vi "PIM Convert 1.0 to 1.1.vi"(0 "PIM 1.0 Test Parameters":T2={"Step Tag"="", "Quickmode?"=FALSE, "PIM Test Stimulus"={"C1 Pwr dBm"=0.0, "C2 Pwr dBm"=0.0, "Power Units"=enum."dBm", "Meas Type"=enum."Band Edges", "C1 Fixed MHz"=0.0, "C2 Fixed MHz"=0.0, "Swept Freq Step"=0}, "Measure"={"IM Order"=0, "Direction"=0, "Averaging"=1, "ALC ON?"=FALSE, "Peak Hold?"=FALSE, "Peak last N"=1, "Ref Level dBm"=-100.0, "Ref Units"=enum."dBm", "Num Samples"=1, "Sample units"=enum."Sample(s)", "Update Rate (s)"=0.0}, "Display"={"Power Scale"={"yRange_min"=-160, "yRange_max"=-60}, "xRange_span"=5}, "Datasheets"={"Datasheets to Generate"=[], "Print Datasheets"=FALSE}} {"Display"."xRange_span" min=5 step=1; "Display"."Power Scale"."yRange_max" min=-200 max=0 step=1; "Display"."Power Scale"."yRange_min" min=-200 max=0 step=1; "Measure"."Update Rate (s)" min=-200.0 max=0.0 step=0.2 format="%.1f"; "Measure"."Num Samples" min=1 max=5000 step=1; "Measure"."Averaging" items=["None", "Minimum", "Normal", "High", "Maximum"]; "Measure"."Ref Level dBm" min=-200.0 max=0.0 step=0.2 format="%.1f"; "Measure"."Peak last N" min=1 max=5000 step=1; "Measure"."Direction" items=["Reverse", "Forward", "Auxiliary"]; "Measure"."IM Order" items=["3rd", "5th", "7th", "9th", "11th", "13th", "15th", "17th", "19th", "21st", "23rd", "25th", "27th", "29th", "31st", "33rd"]; "PIM Test Stimulus"."C2 Fixed MHz" min=-200.0 max=0.0 step=0.2 format="%.1f"; "PIM Test Stimulus"."C1 Fixed MHz" min=-200.0 max=0.0 step=0.2 format="%.1f"; "PIM Test Stimulus"."Swept Freq Step" items=[".2", ".4", "1.0", "2.0"]}) -> (1 "QuickMode":i8, 2 "PIM 1.1 Test Parameters":T1={"PIM Test Stimulus"={"C1 Pwr dBm"=0.0, "C2 Pwr dBm"=0.0, "Power Units"=enum."dBm", "Meas Type"=enum."Band Edges", "C1 Fixed MHz"=0.0, "C2 Fixed MHz"=0.0, "Swept Freq Step"=0}, "Measure"={"IM Order"=0, "Direction"=0, "Averaging"=1, "ALC ON?"=TRUE, "Peak Hold?"=TRUE, "Peak last N"=1, "Ref Level dBm"=-100.0, "Ref Units"=enum."dBm", "Num Samples"=1, "Sample units"=enum."Sample(s)", "Update Rate (s)"=0.0}, "Display"={"Power Scale"={"yRange_min"=0, "yRange_max"=0}, "xRange_span"=5}, "Datasheets"=[]} {"Display"."xRange_span" min=5 step=1; "Display"."Power Scale"."yRange_max" min=-200 max=0 step=1; "Display"."Power Scale"."yRange_min" min=-200 max=0 step=1; "Measure"."Update Rate (s)" min=-200.0 max=0.0 step=0.2 format="%.1f"; "Measure"."Num Samples" min=1 max=5000 step=1; "Measure"."Averaging" items=["None", "Minimum", "Normal", "High", "Maximum"]; "Measure"."Ref Level dBm" min=-200.0 max=0.0 step=0.2 format="%.1f"; "Measure"."Peak last N" min=1 max=5000 step=1; "Measure"."Direction" items=["Reverse", "Forward", "Auxiliary"]; "Measure"."IM Order" items=["3rd", "5th", "7th", "9th", "11th", "13th", "15th", "17th", "19th", "21st", "23rd", "25th", "27th", "29th", "31st", "33rd"]; "PIM Test Stimulus"."C2 Fixed MHz" min=-200.0 max=0.0 step=0.2 format="%.1f"; "PIM Test Stimulus"."C1 Fixed MHz" min=-200.0 max=0.0 step=0.2 format="%.1f"; "PIM Test Stimulus"."Swept Freq Step" items=[".2", ".4", "1.0", "2.0"]})   [LabVIEW 2011]
uses:
  TypeDefs/PIM Test Parameters v1.0.ctl
  TypeDefs/PIM Test Parameters v1.1.ctl
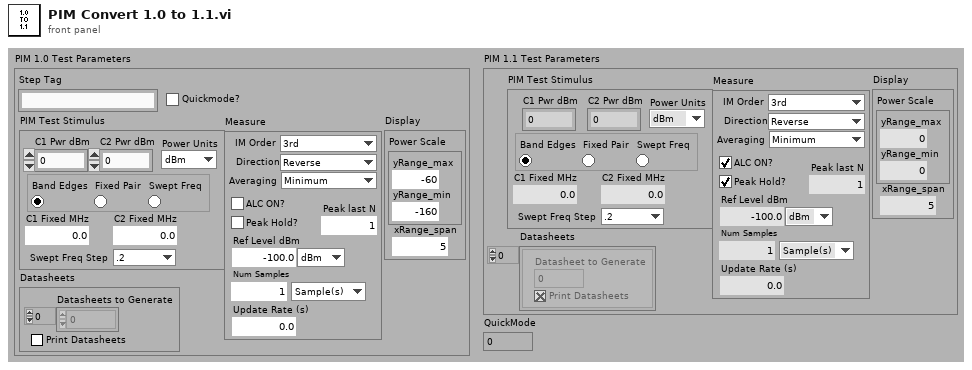
[diagram p1: front panel]
types:
  T1 = typedef "PIM Test Parameters v1.1.ctl" = cluster{"PIM Test Stimulus":cluster{"C1 Pwr dBm":dbl, "C2 Pwr dBm":dbl, "Power Units":enum16{"dBm", "Watts"}, "Meas Type":enum32{"Band Edges", "Fixed Pair", "Swept Freq"}, "C1 Fixed MHz":dbl, "C2 Fixed MHz":dbl, "Swept Freq Step":u16}, "Measure":cluster{"IM Order":u8, "Direction":u16, "Averaging":u16, "ALC ON?":bool, "Peak Hold?":bool, "Peak last N":u32, "Ref Level dBm":dbl, "Ref Units":enum16{"dBm", "dBc"}, "Num Samples":u32, "Sample units":enum16{"Sample(s)", "Second(s)", "Sweep(s)"}, "Update Rate (s)":dbl}, "Display":cluster{"Power Scale":cluster{"yRange_min":i32, "yRange_max":i32}, "xRange_span":u32}, "Datasheets":cluster{"Datasheet to Generate":i32, "Print Datasheets":bool}[]}
  T2 = typedef "PIM Test Parameters v1.0.ctl" = cluster{"Step Tag":string, "Quickmode?":bool, "PIM Test Stimulus":cluster{"C1 Pwr dBm":dbl, "C2 Pwr dBm":dbl, "Power Units":enum16{"dBm", "Watts"}, "Meas Type":enum32{"Band Edges", "Fixed Pair", "Swept Freq"}, "C1 Fixed MHz":dbl, "C2 Fixed MHz":dbl, "Swept Freq Step":u16}, "Measure":cluster{"IM Order":u8, "Direction":u16, "Averaging":u16, "ALC ON?":bool, "Peak Hold?":bool, "Peak last N":u32, "Ref Level dBm":dbl, "Ref Units":enum16{"dBm", "dBc"}, "Num Samples":u32, "Sample units":enum16{"Sample(s)", "Second(s)", "Sweep(s)"}, "Update Rate (s)":dbl}, "Display":cluster{"Power Scale":cluster{"yRange_min":i32, "yRange_max":i32}, "xRange_span":u32}, "Datasheets":cluster{"Datasheets to Generate":i32[], "Print Datasheets":bool}}
  T3 = cluster{"C1 Pwr dBm":dbl, "C2 Pwr dBm":dbl, "Power Units":enum16{"dBm", "Watts"}, "Meas Type":enum32{"Band Edges", "Fixed Pair", "Swept Freq"}, "C1 Fixed MHz":dbl, "C2 Fixed MHz":dbl, "Swept Freq Step":u16}
  T4 = cluster{"IM Order":u8, "Direction":u16, "Averaging":u16, "ALC ON?":bool, "Peak Hold?":bool, "Peak last N":u32, "Ref Level dBm":dbl, "Ref Units":enum16{"dBm", "dBc"}, "Num Samples":u32, "Sample units":enum16{"Sample(s)", "Second(s)", "Sweep(s)"}, "Update Rate (s)":dbl}
  T5 = cluster{"Power Scale":cluster{"yRange_min":i32, "yRange_max":i32}, "xRange_span":u32}
  T6 = cluster{"Datasheet to Generate":i32, "Print Datasheets":bool}[]
  T7 = cluster{"Datasheet to Generate":i32, "Print Datasheets":bool}
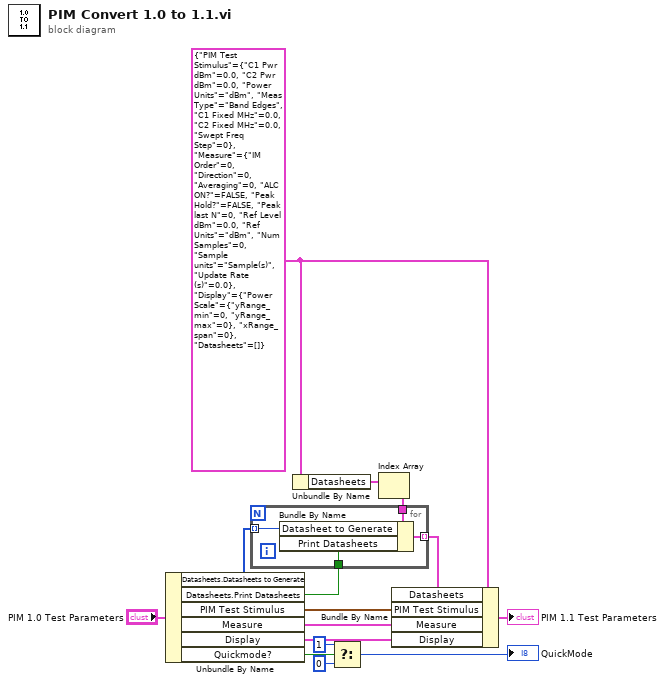
[diagram p0: block diagram]
diagram:
  w13 = T1 {"PIM Test Stimulus"={"C1 Pwr dBm"=0.0, "C2 Pwr dBm"=0.0, "Power Units"=enum."dBm", "Meas Type"=enum."Band Edges", "C1 Fixed MHz"=0.0, "C2 Fixed MHz"=0.0, "Swept Freq Step"=0}, "Measure"={"IM Order"=0, "Direction"=0, "Averaging"=0, "ALC ON?"=FALSE, "Peak Hold?"=FALSE, "Peak last N"=0, "Ref Level dBm"=0.0, "Ref Units"=enum."dBm", "Num Samples"=0, "Sample units"=enum."Sample(s)", "Update Rate (s)"=0.0}, "Display"={"Power Scale"={"yRange_min"=0, "yRange_max"=0}, "xRange_span"=0}, "Datasheets"=[]} ("PIM 1.1 Test Parameters")
  n1 = Unbundle By Name("PIM 1.0 Test Parameters") -> ("Datasheets.Datasheets to Generate"=w5:i32[], "Datasheets.Print Datasheets"=w6:bool, "PIM Test Stimulus"=w7:T3, "Measure"=w8:T4, "Display"=w9:T5, "Quickmode?"=w1:bool)
  n2 = Unbundle By Name(w13) -> ("Datasheets"=w15:T6)
  n3 = Select(t=i8 1 ("QuickMode"), s=w1, f=i8 0 ("QuickMode")) -> (s? t:f=→"QuickMode":i8)
  n4 = Index Array(array=w15) -> (element=w14:T7)  [unwired: 1 in]
  n5 = for {
    tunnel: w14 -> [w19]
    tunnel: [w18] -> w11 mode=indexing
    tunnel: w5 -> [w17] mode=indexing
    tunnel: w6 -> [w16]
    n6 = Bundle By Name(cluster=w19, "Datasheet to Generate"=w17, "Print Datasheets"=w16) -> (w18:T7)
  }
  n7 = Bundle By Name(cluster=w13, "Datasheets"=w11, "PIM Test Stimulus"=w7, "Measure"=w8, "Display"=w9) -> (→"PIM 1.1 Test Parameters":T1)
